vi "SPI Simulation Plotter.vi"(9 "Engine Clock Rate (MHz)":i32=120000000 format="%.0p", 10 "SPI Signals":T2, 11 "SPI PHY Settings":T3={"Divide Value"=10, "Transfer Length (bits)"=24, "CS Asserted Polarity"=FALSE, "Clock Polarity (CPOL)"=FALSE, "Clock Phase (CPHA)"=FALSE, "Lengthen MISO Setup"=FALSE, "Direction Change Bit"=0, "MOSI Starts as Output"=FALSE, "Tristatable MOSI"=FALSE}) -> (2 "Timing Characteristics":T1 {"tCH (ns)" format="%#_4g"; "tCSS (ns)" format="%#_4g"; "tCSH (ns)" format="%#_4g"; "tCSW (ns)" format="%#_4g"; "Actual Sample Rate (Hz)" format="%_4p"; "SCLK Frequency (Hz)" format="%#.2p"}, 3 "Digital Data":digitalwaveform(graph), 5 "Chart Size":i32)   [LabVIEW 2014]
uses:
  Controls/Digital Data.ctl
  Controls/Timing Characteristics.ctl
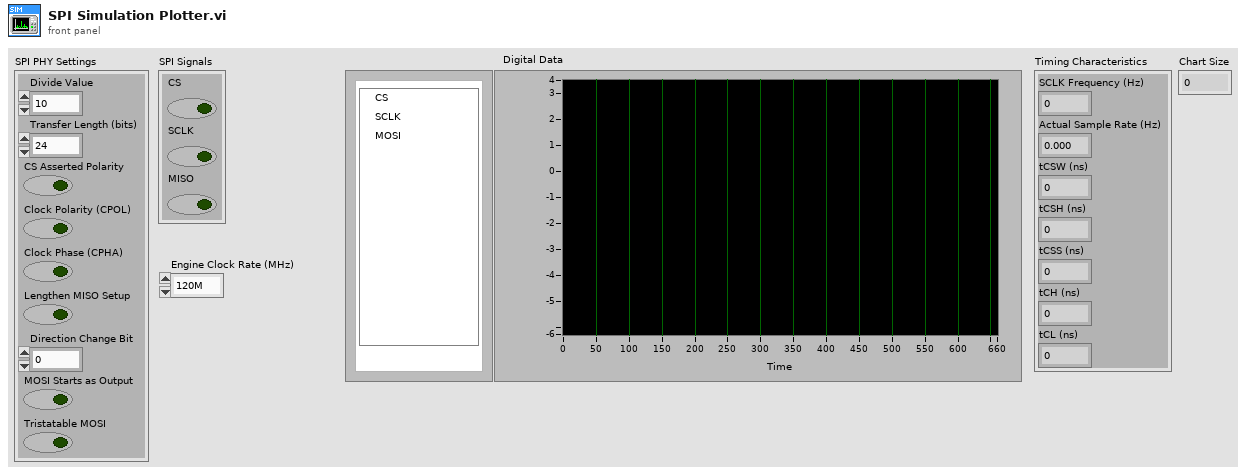
[diagram p1: front panel]
types:
  T1 = typedef "Timing Characteristics.ctl" = cluster{"SCLK Frequency (Hz)":dbl, "Actual Sample Rate (Hz)":dbl, "tCSW (ns)":dbl, "tCSH (ns)":dbl, "tCSS (ns)":dbl, "tCH (ns)":dbl, "tCL (ns)":dbl}
  T2 = typedef "Digital Data.ctl" = cluster{"CS":bool, "SCLK":bool, "MISO":bool}
  T3 = cluster{"Divide Value":u8, "Transfer Length (bits)":u8, "CS Asserted Polarity":bool, "Clock Polarity (CPOL)":bool, "Clock Phase (CPHA)":bool, "Lengthen MISO Setup":bool, "Direction Change Bit":u8, "MOSI Starts as Output":bool, "Tristatable MOSI":bool}
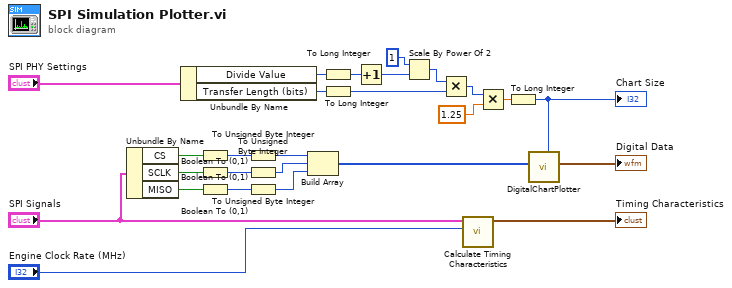
[diagram p0: block diagram]
diagram:
  n1 = Unbundle By Name("SPI Signals") -> ("CS"=w19:bool, "SCLK"=w18:bool, "MISO"=w17:bool)
  n2 = Unbundle By Name("SPI PHY Settings") -> ("Divide Value"=w4:u8, "Transfer Length (bits)"=w5:u8)
  n3 = Boolean To (0,1)(Boolean=w19) -> (0, 1=w15:i16)
  n4 = Boolean To (0,1)(Boolean=w18) -> (0, 1=w14:i16)
  n5 = Boolean To (0,1)(Boolean=w17) -> (0, 1=w13:i16)
  n6 = To Unsigned Byte Integer(number=w15) -> (unsigned 8bit integer=w12:u8)
  n7 = To Unsigned Byte Integer(number=w14) -> (unsigned 8bit integer=w11:u8)
  n8 = To Unsigned Byte Integer(number=w13) -> (unsigned 8bit integer=w10:u8)
  n9 = Build Array(w12, w11, w10) -> (w16:u8[])
  n10 = To Long Integer(number=w4) -> (32bit integer=w3:i32)
  n11 = To Long Integer(number=w5) -> (32bit integer=w2:i32)
  n12 = Increment(x=w3) -> (x+1=w23:i32)
  n13 = Scale By Power Of 2(n=i16 1, x=w23) -> (x*2^n=w22:i32)
  n14 = Multiply(x=w22, y=w2) -> (x*y=w25:i32)
  n15 = call "Calculate Timing Characteristics.vi"("Engine Clock Rate (MHz)"="Engine Clock Rate (MHz)", "SPI Signals"="SPI Signals") -> ("Timing Characteristics"=→"Timing Characteristics":T1)  [unwired: 9 in]
  n16 = Multiply(x=w25, y=1.25 ("History Scale")) -> (x*y=w21:dbl)
  n17 = To Long Integer(number=w21) -> (32bit integer=w8:i32)
  "Chart Size" <- w8
  n18 = call "DigitalChartPlotter.vi"("History Size"=w8, "Input"=w16) -> ("Digital Data"=→"Digital Data":digitalwaveform)  [unwired: 9 in]
